vi "Data.vi"(9 "Run ID":string, 10 "Sample":T1) -> (2 "Message":string)   [LabVIEW 2024, in "Sift Client.lvlib"]
uses:
  Sift Client.lvlib
  Typedefs/Sample.ctl
  Typedefs/Timestamp.ctl
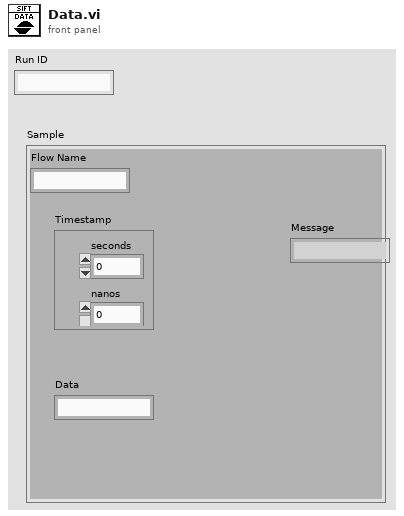
[diagram p1: front panel]
types:
  T1 = typedef "Sift Client.lvlib/Sample.ctl" = cluster{"Flow Name":string, "Timestamp":T2, "Data":string}
  T2 = typedef "Sift Client.lvlib/Timestamp.ctl" = cluster{"seconds":i64, "nanos":i32}
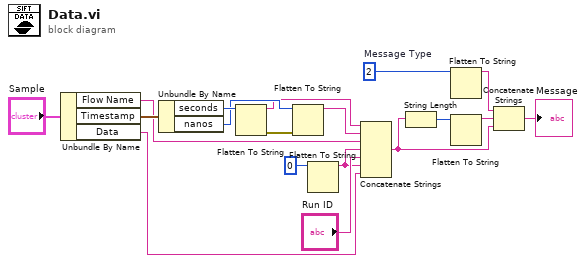
[diagram p0: block diagram]
diagram:
  w13 = u8 2  # Message Type
  n1 = Unbundle By Name("Sample") -> ("Flow Name"=w10:string, "Timestamp"=w17:T2, "Data"=w6:string)
  n2 = Unbundle By Name(w17) -> ("seconds"=w16:i64, "nanos"=w15:i32)
  n3 = Flatten To String(anything=w16) -> (data string=w12:string, error out=w14:errorcluster)  [unwired: 3 in, 1 out]
  n4 = Flatten To String(anything=w15, error in (no error)=w14) -> (data string=w11:string)  [unwired: 2 in, 2 out]
  n5 = Flatten To String(anything=u8 0) -> (data string=w7:string)  [unwired: 3 in, 2 out]
  n6 = Concatenate Strings(w12, w11, w10, w7, "Run ID", w7, w6) -> (w2:string)
  n7 = String Length(string=w2) -> (length=w4:i32)
  n8 = Flatten To String(anything=w13) -> (data string=w5:string)  [unwired: 3 in, 2 out]
  n9 = Flatten To String(anything=w4) -> (data string=w3:string)  [unwired: 3 in, 2 out]
  n10 = Concatenate Strings(w5, w3, w2) -> (→"Message":string)
